vi "UI.vi"(7 "Calculate":bool, 8 "Error In":errorcluster, 9 "B":dbl, 10 "A":dbl, 11 "Data Value Reference In":refnum<data-value>) -> (0 "Error Out":errorcluster, 2 "C":dbl, 3 "Data Value Reference Out":refnum<data-value>)   [LabVIEW 2021, in "Calculator.lvlib" / "Divide.lvclass"]
doc: "This VI is an overriding VI which is opened in subpanel of main VI, which has controls and a boolean button. The user enters the input and the output is displayed in the indicator when calculate is pressed."
uses:
  Divide.lvclass
  Calculator.lvlib
  Controls/User Event Operations.ctl
  NumericOperation/NumericOperation.lvclass
panel:
  # "Divide"
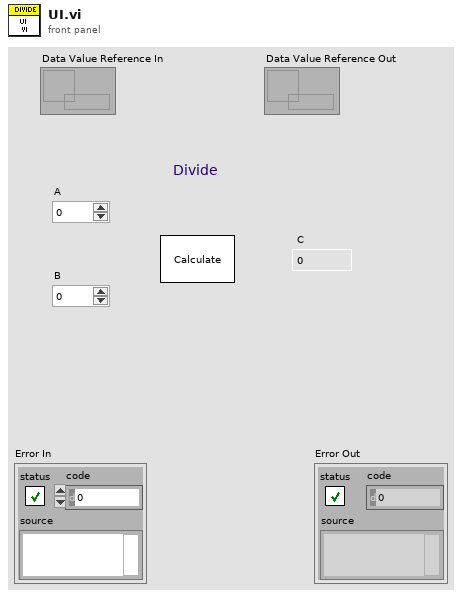
[diagram p1: front panel]
types:
  T1 = typedef "Calculator.lvlib/User Event Operations.ctl" = enum16{"Obtain", "Generate", "Release"}
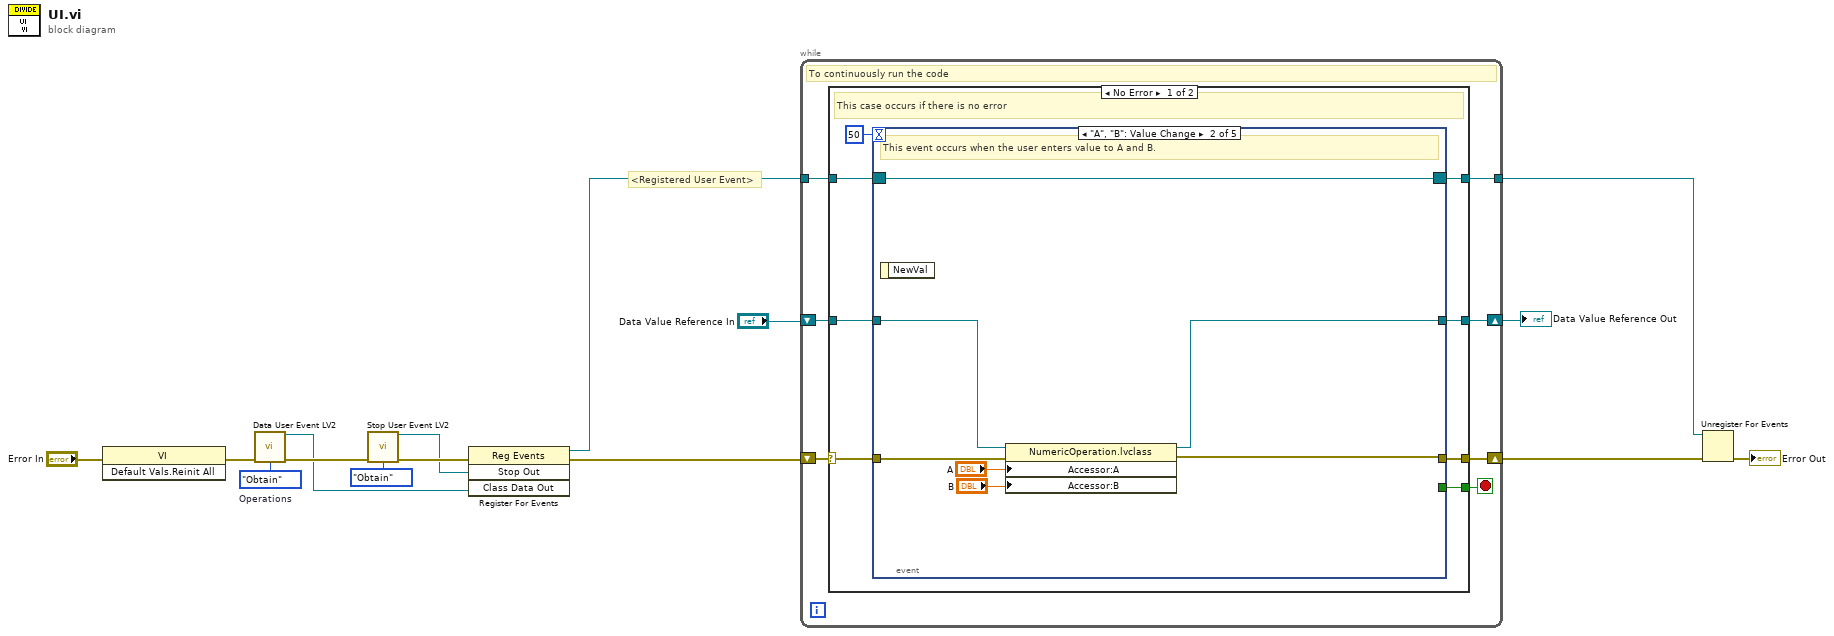
[diagram p0: block diagram]
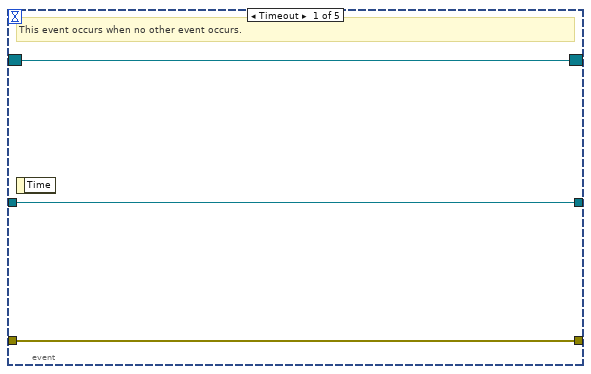
[diagram p2: hidden frame]
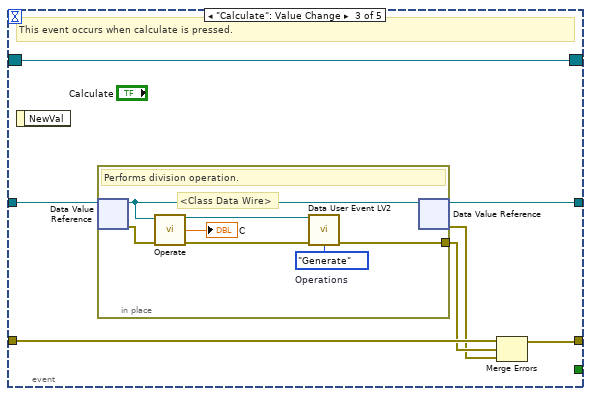
[diagram p3: hidden frame]
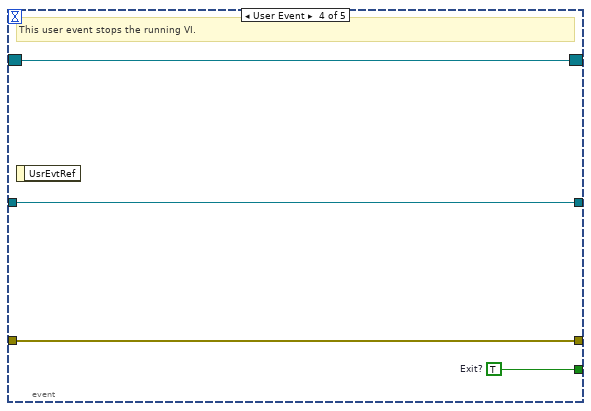
[diagram p4: hidden frame]
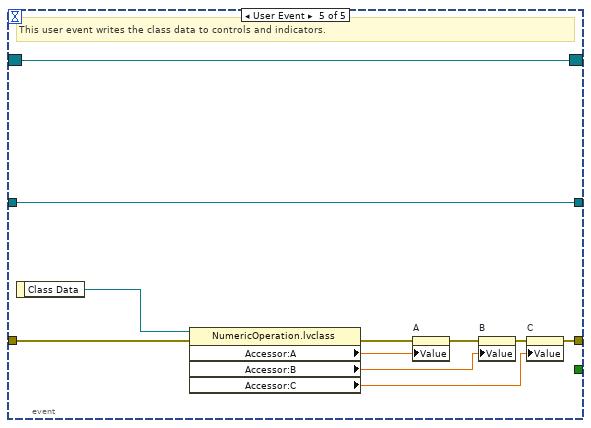
[diagram p5: hidden frame]
diagram:
  w6 = User_Event_Operations."Obtain"  # Operations
  # "<Registered User Event>"
  n1 = invoke class="VI" method="Default Vals.Reinit All"(error in="Error In") -> (error out=w8:errorcluster)  [unwired: 2 in, 2 out]
  n2 = call "Data User Event LV2.vi"("Error In"=w8, "Operations"=w6) -> ("Class Data Out"=w3:refnum<user-event>, "Error Out"=w9:errorcluster)  [unwired: 12 in]
  n3 = call "Stop User Event LV2.vi"("Error In"=w9, "Operations"=User_Event_Operations."Obtain") -> ("Stop Out"=w4:refnum<user-event>, "Error Out"=w7:errorcluster)  [unwired: 12 in]
  n4 = register-events(error in=w7, w4, w3) -> (reference out=w12:refnum<event-registration>, error out=w14:errorcluster)  [unwired: 1 in]
  n5 = while {
    shift-right: [w21] -> w15
    shift-left: w14 -> [w22]
    shift-right: [w19] -> w1
    shift-left: "Data Value Reference In" -> [w20]
    tunnel: w12 -> [w18]
    tunnel: [w16] -> w10
    stop <- w17 stop-if-true
    # "To continuously run the code"
    n6 = case shown="No Error" w22 {
      selector: w22 -> [w25 w72]
      tunnel: [w24 w72] -> w21
      tunnel: [w29 w71] -> w19
      tunnel: w20 -> [w30 w71]
      tunnel: w18 -> [w27 w70]
      tunnel: [w26 _] -> w17
      tunnel: [w23 w70] -> w16
      frame No Error {
        # "This case occurs if there is no error"
        n7 = event shown="[1] \"A\", \"B\": Value Change" {
          selector: w27 -> [w31 w34 w47 w55 w59]
          dyn-events: [w31 w34 w47 w55 w59] -> w23
          timeout: 50 -> [_ _ _ _ _]
          tunnel: [w33 w35 w44 w57 w60] -> w29
          tunnel: w30 -> [w33 w40 w45 w57 w60]
          tunnel: [_ _ _ w58 _] -> w26
          tunnel: [w32 w36 w41 w56 w63] -> w24
          tunnel: w25 -> [w32 w39 w46 w56 w69]
          event Timeout {
            # "This event occurs when no other event occurs."
            n8 = event-data() -> ()  [unwired: 1 in, 1 out]
          }
          event "A", "B": Value Change {
            # "This event occurs when the user enters value to A and B."
            n9 = event-data() -> ()  [unwired: 1 in, 1 out]
            n10 = property class="NumericOperation.lvclass"(reference=w40, error in=w39, "Accessor:A"="A", "Accessor:B"="B") -> (reference out=w35:refnum<data-value>, error out=w36:errorcluster)
          }
          event "Calculate": Value Change {
            # "This event occurs when calculate is pressed."
            n11 = event-data() -> ()  [unwired: 1 in, 1 out]
            n12 = in-place {
              in-place-border: [w52] -> w43
              w51 = User_Event_Operations."Generate"  # Operations
              # "<Class Data Wire>"
              # "Performs division operation."
              n13 = in-place-dvr #1(w45) -> (w48:refnum<class "NumericOperation.lvclass">, w49:errorcluster)
              n14 = call-dynamic "Operate.vi"("Error In"=w49, "NumericOperation in"=w48) -> ("Error Out"=w53:errorcluster, "C"=→"C":dbl, "NumericOperation out"=w50:refnum<class "NumericOperation.lvclass">)  [unwired: 7 in]
              n15 = call "Data User Event LV2.vi"("Class Data"=w50, "Error In"=w53, "Operations"=w51) -> ("Error Out"=w52:errorcluster)  [unwired: 11 in, 1 out]
              n16 = in-place-dvr #1(w48) -> (w44:refnum<data-value>, w42:errorcluster)
            }
            n17 = Merge Errors(w46, w43, w42) -> (w41:errorcluster)
          }
          event User Event {
            w58 = TRUE  # Exit?
            # "This user event stops the running VI."
            n18 = event-data() -> ()  [unwired: 1 in, 1 out]
          }
          event User Event {
            # "This user event writes the class data to controls and indicators."
            n19 = event-data() -> ("Class Data"=w66:refnum<class "NumericOperation.lvclass">)  [unwired: 1 in]
            n20 = property class="NumericOperation.lvclass"(reference=w66, error in=w69) -> (error out=w68:errorcluster, "Accessor:A"=w65:dbl, "Accessor:B"=w62:dbl, "Accessor:C"=w61:dbl)  [unwired: 1 out]
            n21 = property on="A" class="DigNum (strict)"(error in=w68, "Value"=w65) -> (error out=w67:errorcluster)  [unwired: 1 in, 1 out]
            n22 = property on="B" class="DigNum (strict)"(error in=w67, "Value"=w62) -> (error out=w64:errorcluster)  [unwired: 1 in, 1 out]
            n23 = property on="C" class="DigNum (strict)"(error in=w64, "Value"=w61) -> (error out=w63:errorcluster)  [unwired: 1 in, 1 out]
          }
        }
      }
      frame Error {
        # "This case occurs if there is any error."
      }
    }
  }
  "Data Value Reference Out" <- w1
  n24 = Unregister For Events(event registration refnum=w10, error in=w15) -> (error out=→"Error Out":errorcluster)
